vi "Module ID.vi"(11 "GUI Manager Module in":refnum<class "GUI Manager Module.lvclass">) -> (2 "Module ID":string)   [LabVIEW 2020, in "VolatusGUI.lvlib" / "GUI Manager Module.lvclass"]
uses:
  GUI Manager Module.lvclass
  GUI Manager Module.lvclass/GUI Manager Module.ctl
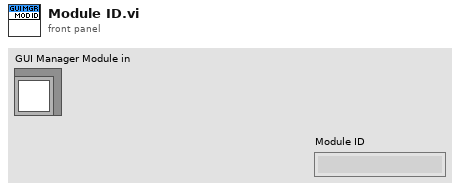
[diagram p1: front panel]
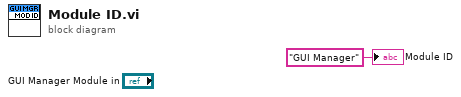
[diagram p0: block diagram]
diagram:
  "Module ID" <- "GUI Manager" ("Module ID")
